vi "SetupSweepAndGetPeak.vi"(6 "Route Names":string[](array[string]), 7 "Cal?":bool, 8 "error in (no error)":errorcluster, 9 "Span(Hz)":dbl=26500000000.0, 10 "Center Frequency(Hz)":dbl=13250000000.0, 11 "NetA_RSZVL in":refnum<class "NetA_RSZVL.lvclass">) -> (0 "error out":errorcluster, 1 "FDelta(hz)":dbl, 2 "Calibrated Amplitude (dBm)":dbl, 3 "NetA_RSZVL out":refnum<class "NetA_RSZVL.lvclass">)   [LabVIEW 2014, in "NetA_RSZVL.lvclass"]
uses:
  NetA_RSZVL.lvclass
  NetA_RSZVL.lvclass/NetA_RSZVL.ctl
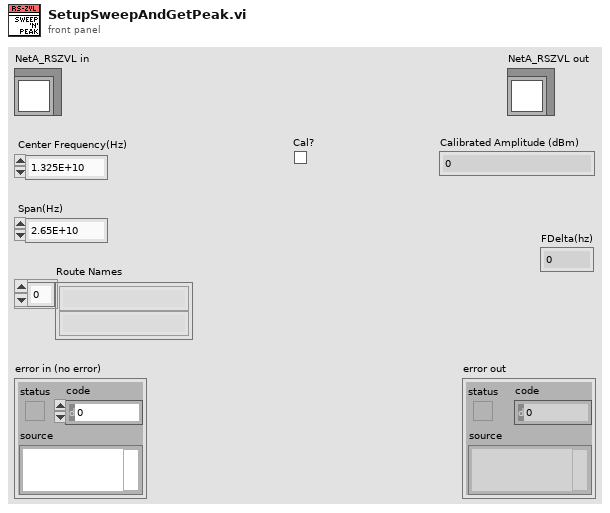
[diagram p1: front panel]
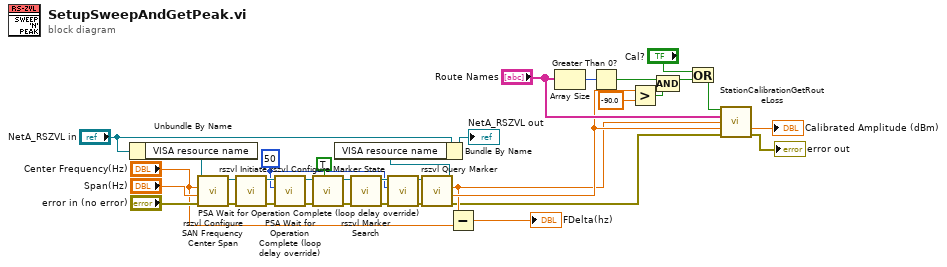
[diagram p0: block diagram]
diagram:
  w4 = u32 50 ("loop delay (ms)")
  n1 = Unbundle By Name("NetA_RSZVL in") -> ("VISA resource name"=w33:refnum<visa-resource-name>)
  n2 = call "rszvl Configure SAN Frequency Center Span.vi"("error in (no error)"="error in (no error)", "Span"="Span(Hz)", "Center Frequency"="Center Frequency(Hz)", "VISA resource name"=w33) -> ("error out"=w29:errorcluster, "VISA resource name out"=w30:refnum<visa-resource-name>)  [unwired: 6 in]
  n3 = call "rszvl Initiate.vi"("error in (no error)"=w29, "VISA resource name"=w30) -> ("error out"=w21:errorcluster, "VISA resource name out"=w22:refnum<visa-resource-name>)  [unwired: 8 in]
  n4 = call "PSA Wait for Operation Complete (loop delay override).vi"("error in (no error)"=w21, "loop delay (ms)"=w4, "VISA resource name"=w22) -> ("error out"=w19:errorcluster, "VISA resource name out"=w20:refnum<visa-resource-name>)  [unwired: 7 in]
  n5 = call "rszvl Configure Marker State.vi"("Marker State (Off)"=TRUE, "error in (no error)"=w19, "VISA resource name"=w20) -> ("error out"=w26:errorcluster, "VISA resource name out"=w27:refnum<visa-resource-name>)  [unwired: 7 in]
  n6 = call "rszvl Marker Search.vi"("error in (no error)"=w26, "VISA resource name"=w27) -> ("error out"=w8:errorcluster, "VISA resource name out"=w7:refnum<visa-resource-name>)  [unwired: 8 in]
  n7 = call "PSA Wait for Operation Complete (loop delay override).vi"("error in (no error)"=w8, "loop delay (ms)"=w4, "VISA resource name"=w7) -> ("error out"=w5:errorcluster, "VISA resource name out"=w6:refnum<visa-resource-name>)  [unwired: 7 in]
  n8 = call "rszvl Query Marker.vi"("error in (no error)"=w5, "VISA resource name"=w6) -> ("error out"=w9:errorcluster, "Marker Amplitude"=w13:dbl, "Marker Position"=w12:dbl, "VISA resource name out"=w23:refnum<visa-resource-name>)  [unwired: 6 in]
  n9 = Bundle By Name(cluster="NetA_RSZVL in", "VISA resource name"=w23) -> (→"NetA_RSZVL out":refnum<class "NetA_RSZVL.lvclass">)
  n10 = Subtract(x=w12, y="Center Frequency(Hz)") -> (x-y=→"FDelta(hz)":dbl)
  n11 = Array Size(array="Route Names") -> (size(s)=w17:i32)
  n12 = Greater Than 0?(x=w17) -> (x > 0?=w15:bool)
  n13 = Greater?(x=w13, y=-90.0) -> (0:w16:bool)
  n14 = Compound Arithmetic op=AND(w15, w16) -> (w2:bool)
  n15 = Or(x="Cal?", y=w2) -> (x .or. y?=w3:bool)
  n16 = call "StationCalibrationGetRouteLoss.vi"("Calibration Enabled"=w3, "Route Names"="Route Names", "Frequency"=w12, "Power Level"=w13, "error in (no error)"=w9) -> ("Adjusted Power Level"=→"Calibrated Amplitude (dBm)":dbl, "error out"=→"error out":errorcluster)  [unwired: 7 in, 2 out]
